vi "Right Motor Control Loop (SubVI).vi"   [LabVIEW 2015]
uses:
  Right Variables.vi
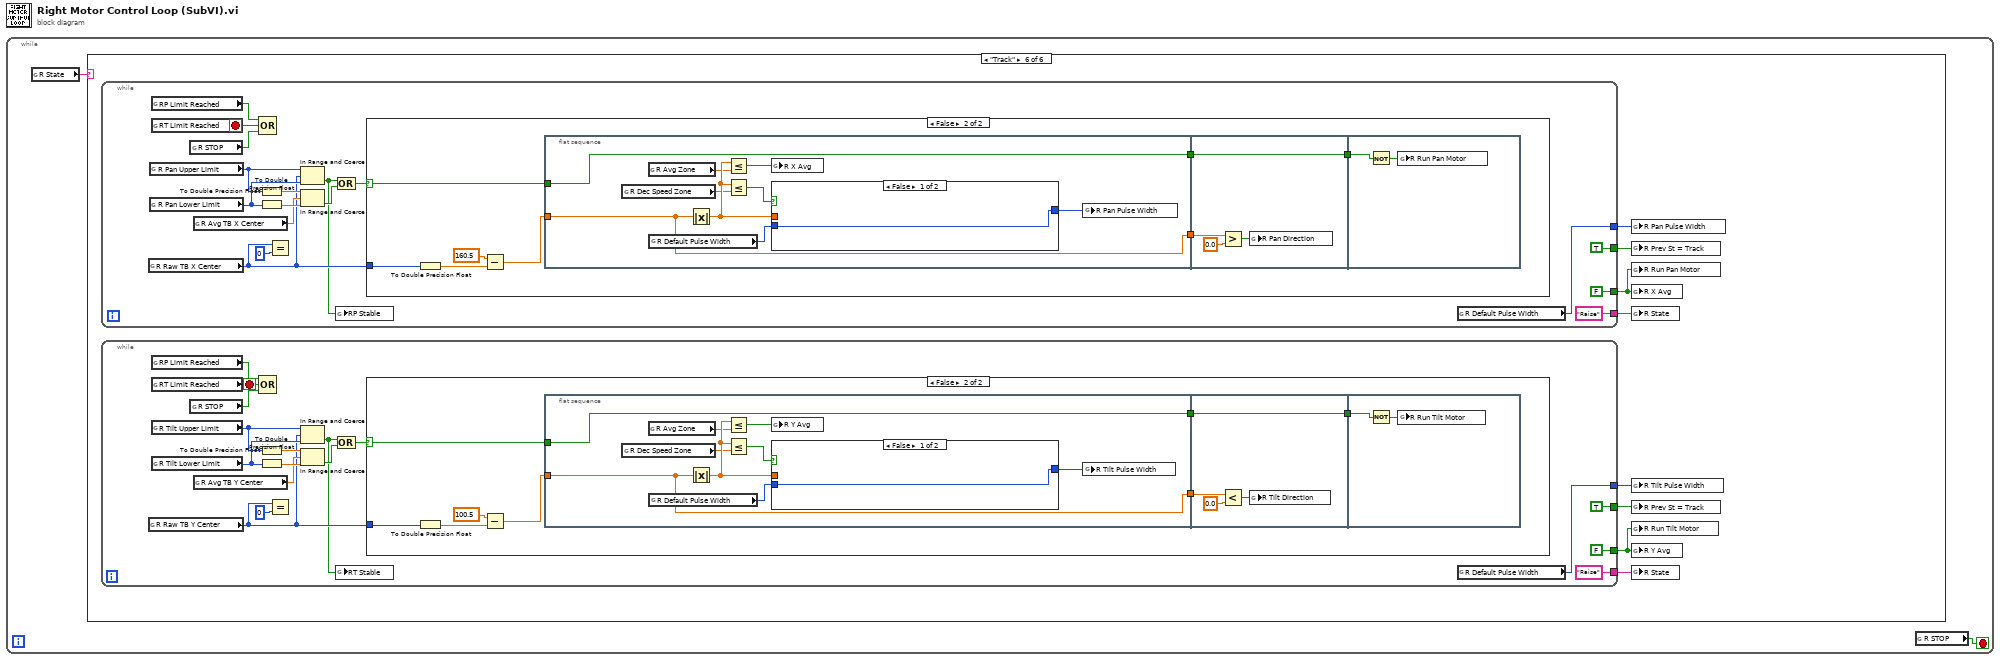
[diagram p0: block diagram]
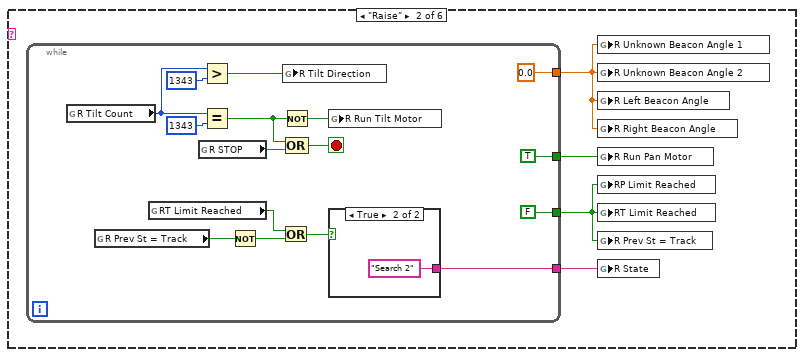
[diagram p3: hidden frame]
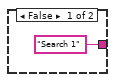
[diagram p4: hidden frame]
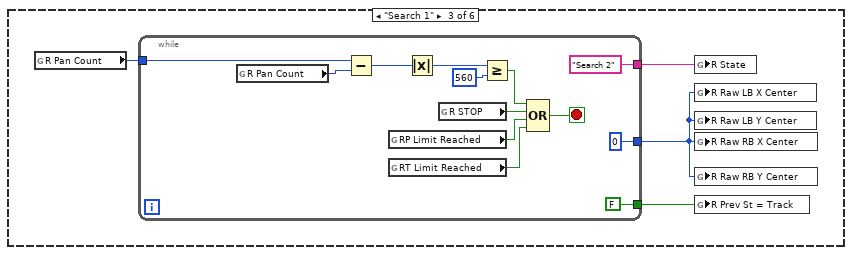
[diagram p5: hidden frame]
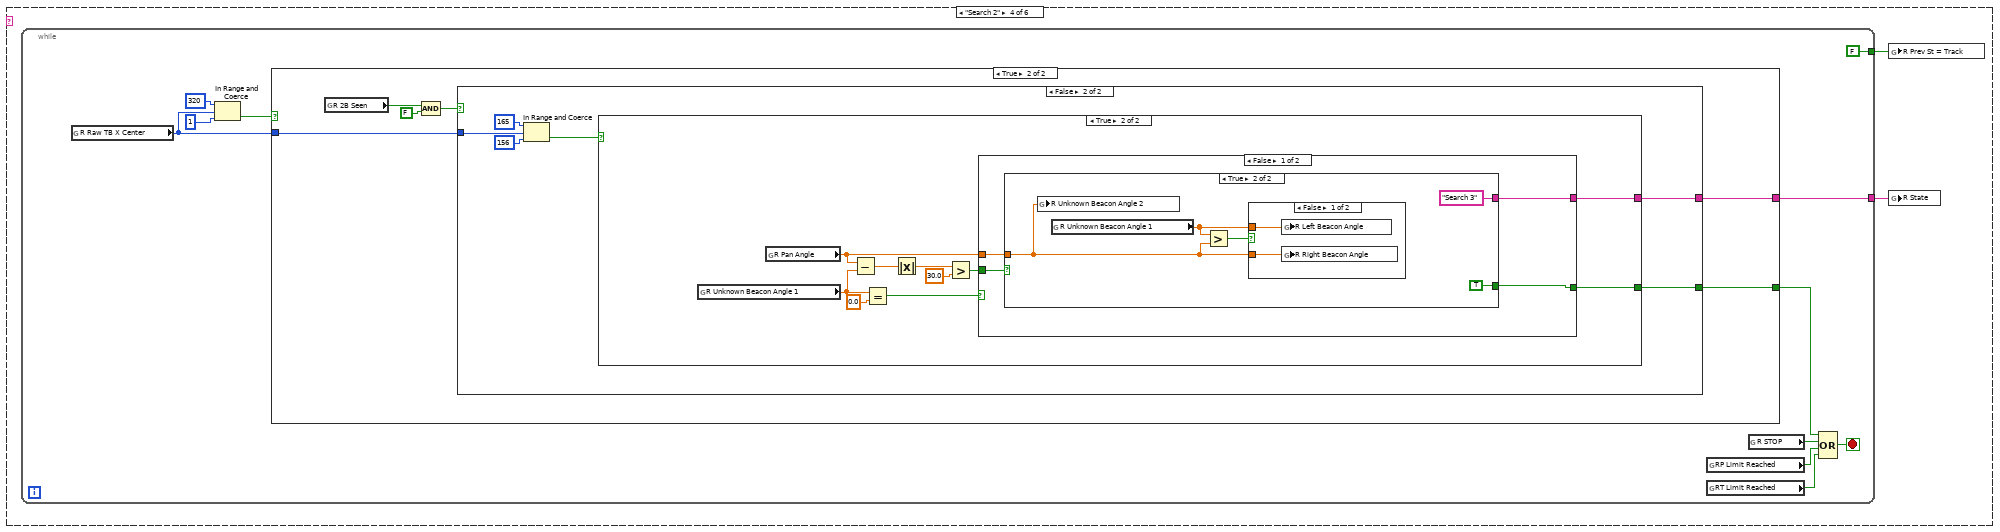
[diagram p6: hidden frame]
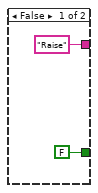
[diagram p7: hidden frame]
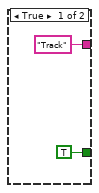
[diagram p8: hidden frame]
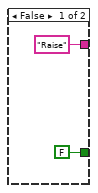
[diagram p9: hidden frame]
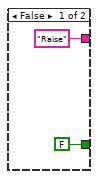
[diagram p10: hidden frame]
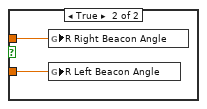
[diagram p11: hidden frame]
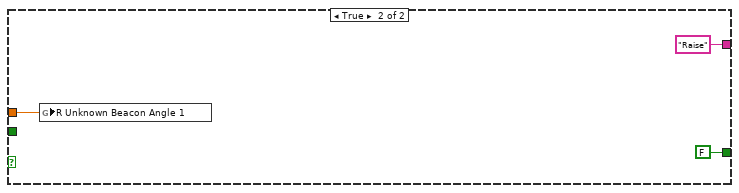
[diagram p12: hidden frame]
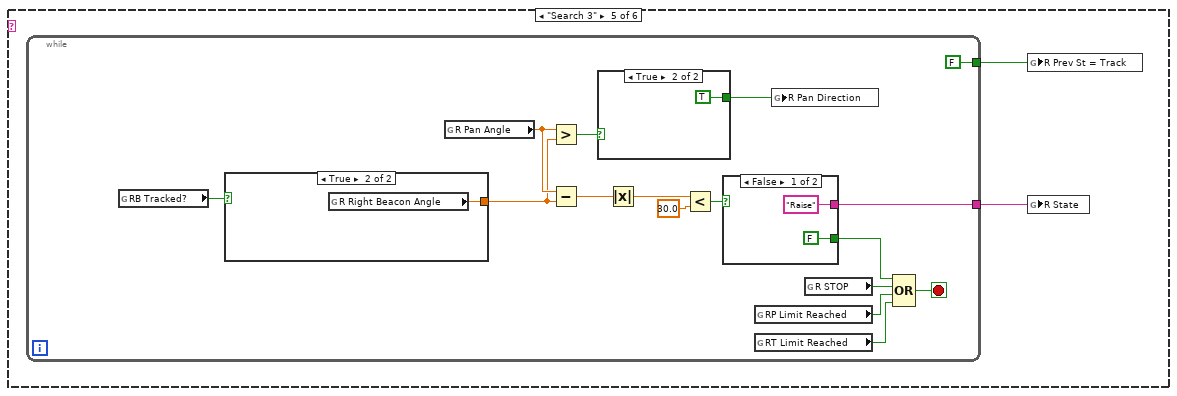
[diagram p13: hidden frame]
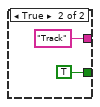
[diagram p14: hidden frame]
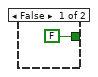
[diagram p15: hidden frame]
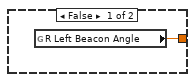
[diagram p16: hidden frame]
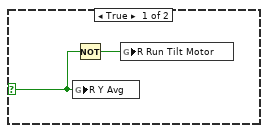
[diagram p17: hidden frame]
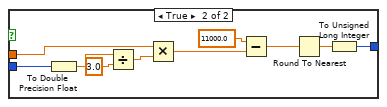
[diagram p18: hidden frame]
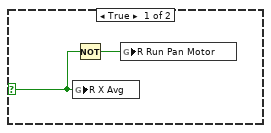
[diagram p19: hidden frame]
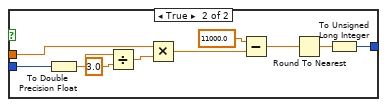
[diagram p20: hidden frame]
diagram:
  n1 = while {
    stop <- w1 stop-if-true
    n2 = global read "Right Variables.vi" "R State"() -> (w2:string)
    n3 = case shown="\"Track\"" w2 {
      frame "Null", Default {
      }
      frame "Raise" {
        n4 = while {
          tunnel: [w21] -> w6
          tunnel: [FALSE] -> w3
          tunnel: [TRUE ("L Run Pan Motor")] -> w5
          tunnel: [0.0] -> w4
          stop <- w22 stop-if-true
          n5 = global read "Right Variables.vi" "R Tilt Count"() -> (w17:i32)
          n6 = global read "Right Variables.vi" "R Prev St = Track"() -> (w10:bool)
          n7 = global read "Right Variables.vi" "RT Limit Reached"() -> (w8:bool)
          n8 = global read "Right Variables.vi" "R STOP"() -> (w14:bool)
          n9 = Greater?(x=w17, y=1343) -> (0:w15:bool)
          n10 = Equal?(x=w17, y=1343) -> (x = y?=w18:bool)
          n11 = Not(x=w10) -> (.not. x?=w9:bool)
          n12 = Or(x=w8, y=w9) -> (x .or. y?=w7:bool)
          n13 = Not(x=w18) -> (.not. x?=w16:bool)
          n14 = global write "Right Variables.vi" "R Tilt Direction"(w15) -> ()
          n15 = Compound Arithmetic op=OR(w18, w14) -> (w22:bool)
          n16 = global write "Right Variables.vi" "R Run Tilt Motor"(w16) -> ()
          n17 = case shown="True" w7 {
            tunnel: ["Search 1" ("L State") "Search 2" ("L State")] -> w21
            frame False {
            }
            frame True {
            }
          }
        }
        n18 = global write "Right Variables.vi" "R Unknown Beacon Angle 1"(w4) -> ()
        n19 = global write "Right Variables.vi" "R Unknown Beacon Angle 2"(w4) -> ()
        n20 = global write "Right Variables.vi" "R Left Beacon Angle"(w4) -> ()
        n21 = global write "Right Variables.vi" "R Right Beacon Angle"(w4) -> ()
        n22 = global write "Right Variables.vi" "R Run Pan Motor"(w5) -> ()
        n23 = global write "Right Variables.vi" "RP Limit Reached"(w3) -> ()
        n24 = global write "Right Variables.vi" "RT Limit Reached"(w3) -> ()
        n25 = global write "Right Variables.vi" "R Prev St = Track"(w3) -> ()
        n26 = global write "Right Variables.vi" "R State"(w6) -> ()
      }
      frame "Search 1" {
        n27 = global read "Right Variables.vi" "R Pan Count"() -> (w28:i32)
        n28 = while {
          tunnel: ["Search 2"] -> w27
          tunnel: w28 -> [w37]
          tunnel: [u16 0] -> w26
          tunnel: [FALSE] -> w25
          stop <- w41 stop-if-true
          n29 = global read "Right Variables.vi" "R Pan Count"() -> (w34:i32)
          n30 = Subtract(x=w37, y=w34) -> (x-y=w36:i32)
          n31 = global read "Right Variables.vi" "RP Limit Reached"() -> (w31:bool)
          n32 = global read "Right Variables.vi" "RT Limit Reached"() -> (w30:bool)
          n33 = Absolute Value(x=w36) -> (abs(x)=w35:i32)
          n34 = global read "Right Variables.vi" "R STOP"() -> (w33:bool)
          n35 = Greater Or Equal?(x=w35, y=560) -> (x >= y?=w38:bool)
          n36 = Compound Arithmetic op=OR(w38, w33, w31, w30) -> (w41:bool)
        }
        n37 = global write "Right Variables.vi" "R State"(w27) -> ()
        n38 = global write "Right Variables.vi" "R Raw LB X Center"(w26) -> ()
        n39 = global write "Right Variables.vi" "R Raw LB Y Center"(w26) -> ()
        n40 = global write "Right Variables.vi" "R Raw RB X Center"(w26) -> ()
        n41 = global write "Right Variables.vi" "R Raw RB Y Center"(w26) -> ()
        n42 = global write "Right Variables.vi" "R Prev St = Track"(w25) -> ()
      }
      frame "Search 2" {
        n43 = while {
          tunnel: [w48] -> w43
          tunnel: [FALSE] -> w42
          stop <- w52 stop-if-true
          n44 = global read "Right Variables.vi" "R Raw TB X Center"() -> (w49:u16)
          n45 = In Range and Coerce(upper limit=u16 320, x=w49, lower limit=u16 1) -> (In Range?=w50:bool)  [unwired: 1 out]
          n46 = case shown="True" w50 {
            tunnel: w49 -> [_ w62]
            tunnel: ["Raise" w61] -> w48
            tunnel: [FALSE w60] -> w47
            frame False {
            }
            frame True {
              n47 = global read "Right Variables.vi" "R 2B Seen"() -> (w59:bool)
              n48 = Compound Arithmetic op=AND(w59, FALSE ("y")) -> (w57:bool)
              n49 = case shown="False" w57 {
                tunnel: w62 -> [_ w70]
                tunnel: ["Track" w66] -> w61
                tunnel: [TRUE w67] -> w60
                frame True {
                }
                frame False {
                  n50 = In Range and Coerce(upper limit=u16 165, x=w70, lower limit=u16 156) -> (In Range?=w68:bool)  [unwired: 1 out]
                  n51 = case shown="True" w68 {
                    tunnel: [FALSE w76] -> w67
                    tunnel: ["Raise" w74] -> w66
                    frame False {
                    }
                    frame True {
                      n52 = global read "Right Variables.vi" "R Unknown Beacon Angle 1"() -> (w75:dbl)
                      n53 = global read "Right Variables.vi" "R Pan Angle"() -> (w73:dbl)
                      n54 = Subtract(x=w73, y=w75) -> (x-y=w81:dbl)
                      n55 = Equal?(x=w75, y=0.0) -> (x = y?=w78:bool)
                      n56 = Absolute Value(x=w81) -> (abs(x)=w80:dbl)
                      n57 = Greater?(x=w80, y=30.0) -> (0:w77:bool)
                      n58 = case shown="False" w78 {
                        tunnel: w73 -> [w86 w99]
                        tunnel: w77 -> [w85 _]
                        tunnel: [w84 FALSE] -> w76
                        tunnel: [w83 "Raise"] -> w74
                        frame False {
                          n59 = case shown="True" w85 {
                            tunnel: w86 -> [_ w89]
                            tunnel: [FALSE TRUE] -> w84
                            tunnel: ["Raise" "Search 3"] -> w83
                            frame False {
                            }
                            frame True {
                              n60 = global write "Right Variables.vi" "R Unknown Beacon Angle 2"(w89) -> ()
                              n61 = global read "Right Variables.vi" "R Unknown Beacon Angle 1"() -> (w91:dbl)
                              n62 = Greater?(x=w91, y=w89) -> (0:w93:bool)
                              n63 = case shown="False" w93 {
                                tunnel: w91 -> [w95 w97]
                                tunnel: w89 -> [w94 w96]
                                frame False {
                                n64 = global write "Right Variables.vi" "R Left Beacon Angle"(w95) -> ()
                                n65 = global write "Right Variables.vi" "R Right Beacon Angle"(w94) -> ()
                                }
                                frame True {
                                n66 = global write "Right Variables.vi" "R Right Beacon Angle"(w97) -> ()
                                n67 = global write "Right Variables.vi" "R Left Beacon Angle"(w96) -> ()
                                }
                              }
                            }
                          }
                        }
                        frame True {
                          n68 = global write "Right Variables.vi" "R Unknown Beacon Angle 1"(w99) -> ()
                        }
                      }
                    }
                  }
                }
              }
            }
          }
          n69 = global read "Right Variables.vi" "RP Limit Reached"() -> (w46:bool)
          n70 = global read "Right Variables.vi" "RT Limit Reached"() -> (w45:bool)
          n71 = global read "Right Variables.vi" "R STOP"() -> (w51:bool)
          n72 = Compound Arithmetic op=OR(w47, w51, w46, w45) -> (w52:bool)
        }
        n73 = global write "Right Variables.vi" "R Prev St = Track"(w42) -> ()
        n74 = global write "Right Variables.vi" "R State"(w43) -> ()
      }
      frame "Search 3" {
        n75 = while {
          tunnel: [w104] -> w102
          tunnel: [FALSE] -> w101
          stop <- w109 stop-if-true
          n76 = global read "Right Variables.vi" "RB Tracked?"() -> (w118:bool)
          n77 = case shown="True" w118 {
            tunnel: [w125 w126] -> w114
            frame False {
              n78 = global read "Right Variables.vi" "R Left Beacon Angle"() -> (w125:dbl)
            }
            frame True {
              n79 = global read "Right Variables.vi" "R Right Beacon Angle"() -> (w126:dbl)
            }
          }
          n80 = global read "Right Variables.vi" "R Pan Angle"() -> (w115:dbl)
          n81 = Greater?(x=w115, y=w114) -> (0:w117:bool)
          n82 = Subtract(x=w115, y=w114) -> (x-y=w106:dbl)
          n83 = case shown="True" w117 {
            tunnel: [FALSE TRUE] -> w116
            frame False {
            }
            frame True {
            }
          }
          n84 = Absolute Value(x=w106) -> (abs(x)=w105:dbl)
          n85 = Less?(x=w105, y=30.0) -> (x < y?=w112:bool)
          n86 = case shown="False" w112 {
            tunnel: ["Raise" "Track"] -> w104
            tunnel: [FALSE TRUE] -> w111
            frame False {
            }
            frame True {
            }
          }
          n87 = global read "Right Variables.vi" "RP Limit Reached"() -> (w108:bool)
          n88 = global read "Right Variables.vi" "RT Limit Reached"() -> (w107:bool)
          n89 = global write "Right Variables.vi" "R Pan Direction"(w116) -> ()
          n90 = global read "Right Variables.vi" "R STOP"() -> (w110:bool)
          n91 = Compound Arithmetic op=OR(w111, w110, w108, w107) -> (w109:bool)
        }
        n92 = global write "Right Variables.vi" "R Prev St = Track"(w101) -> ()
        n93 = global write "Right Variables.vi" "R State"(w102) -> ()
      }
      frame "Track" {
        n94 = while {
          tunnel: ["Raise"] -> w134
          tunnel: [FALSE] -> w131
          tunnel: [TRUE] -> w130
          tunnel: [w189] -> w128
          stop <- w206 stop-if-true
          n95 = global read "Right Variables.vi" "R Raw TB X Center"() -> (w194:u16)
          n96 = global read "Right Variables.vi" "R Pan Upper Limit"() -> (w201:u16)
          n97 = global read "Right Variables.vi" "R Pan Lower Limit"() -> (w200:u16)
          n98 = global read "Right Variables.vi" "RP Limit Reached"() -> (w196:bool)
          n99 = global read "Right Variables.vi" "RT Limit Reached"() -> (w198:bool)
          n100 = global read "Right Variables.vi" "R STOP"() -> (w197:bool)
          n101 = global read "Right Variables.vi" "R Avg TB X Center"() -> (w199:dbl)
          n102 = Compound Arithmetic op=OR(w196, w198, w197) -> (w206:bool)
          n103 = To Double Precision Float(number=w201) -> (double precision float=w204:dbl)
          n104 = To Double Precision Float(number=w200) -> (double precision float=w203:dbl)
          n105 = Equal?(x=w194, y=u16 0) -> ()  [unwired: 1 out]
          n106 = In Range and Coerce(upper limit=w201, x=w194, lower limit=w200) -> (In Range?=w192:bool)  [unwired: 1 out]
          n107 = In Range and Coerce(upper limit=w204, x=w199, lower limit=w203) -> (In Range?=w202:bool)  [unwired: 1 out]
          n108 = global write "Right Variables.vi" "RP Stable"(w192) -> ()
          n109 = Compound Arithmetic op=OR(w192, w202) -> (w191:bool)
          n110 = case shown="False" w191 {
            selector: w191 -> [w208 w209]
            tunnel: w194 -> [_ w216]
            frame True {
              n111 = global write "Right Variables.vi" "R X Avg"(w208) -> ()
              n112 = Not(x=w208) -> (.not. x?=w207:bool)
              n113 = global write "Right Variables.vi" "R Run Pan Motor"(w207) -> ()
            }
            frame False {
              n114 = To Double Precision Float(number=w216) -> (double precision float=w214:dbl)
              n115 = Subtract(x=160.5, y=w214) -> (x-y=w213:dbl)
              n116 = flat-sequence {
                tunnel: w213 -> [w218]
                tunnel: [w218] -> w212
                tunnel: [w217] -> w210
                tunnel: w209 -> [w217]
                tunnel: w212 -> [w238]
                tunnel: [w237] -> w211
                tunnel: w210 -> [w237]
                tunnel: w211 -> [w241]
                frame #0 {
                  n117 = global read "Right Variables.vi" "R Dec Speed Zone"() -> (w222:dbl)
                  n118 = global read "Right Variables.vi" "R Avg Zone"() -> (w223:dbl)
                  n119 = global read "Right Variables.vi" "R Default Pulse Width"() -> (w221:u32)
                  n120 = Absolute Value(x=w218) -> (abs(x)=w224:dbl)
                  n121 = Less Or Equal?(x=w224, y=w223) -> (x <= y?=w220:bool)
                  n122 = Less Or Equal?(x=w224, y=w222) -> (x <= y?=w225:bool)
                  n123 = global write "Right Variables.vi" "R X Avg"(w220) -> ()
                  n124 = case shown="False" w225 {
                    tunnel: w221 -> [w226 w236]
                    tunnel: [w226 w229] -> w219
                    tunnel: w224 -> [_ w227]
                    frame False {
                    }
                    frame True {
                      n125 = To Double Precision Float(number=w236) -> (double precision float=w228:dbl)
                      n126 = Divide(x=w228, y=3.0) -> (x/y=w233:dbl)
                      n127 = Multiply(x=w227, y=w233) -> (x*y=w232:dbl)
                      n128 = Subtract(x=11000.0, y=w232) -> (x-y=w231:dbl)
                      n129 = Round To Nearest(number=w231) -> (nearest integer value=w230:dbl)
                      n130 = To Unsigned Long Integer(number=w230) -> (unsigned 32bit integer=w229:u32)
                    }
                  }
                  n131 = global write "Right Variables.vi" "R Pan Pulse Width"(w219) -> ()
                }
                frame #1 {
                  n132 = Greater?(x=w238, y=0.0) -> (0:w240:bool)
                  n133 = global write "Right Variables.vi" "R Pan Direction"(w240) -> ()
                }
                frame #2 {
                  n134 = Not(x=w241) -> (.not. x?=w242:bool)
                  n135 = global write "Right Variables.vi" "R Run Pan Motor"(w242) -> ()
                }
              }
            }
          }
          n136 = global read "Right Variables.vi" "R Default Pulse Width"() -> (w189:u32)
        }
        n137 = while {
          tunnel: ["Raise"] -> w133
          tunnel: [FALSE] -> w132
          tunnel: [TRUE] -> w129
          tunnel: [w135] -> w127
          stop <- w152 stop-if-true
          n138 = global read "Right Variables.vi" "R Raw TB Y Center"() -> (w139:u16)
          n139 = global read "Right Variables.vi" "RP Limit Reached"() -> (w142:bool)
          n140 = global read "Right Variables.vi" "RT Limit Reached"() -> (w146:bool)
          n141 = global read "Right Variables.vi" "R Tilt Upper Limit"() -> (w145:u16)
          n142 = global read "Right Variables.vi" "R Tilt Lower Limit"() -> (w144:u16)
          n143 = global read "Right Variables.vi" "R STOP"() -> (w147:bool)
          n144 = global read "Right Variables.vi" "R Avg TB Y Center"() -> (w143:dbl)
          n145 = Compound Arithmetic op=OR(w142, w146, w147) -> (w152:bool)
          n146 = To Double Precision Float(number=w145) -> (double precision float=w150:dbl)
          n147 = To Double Precision Float(number=w144) -> (double precision float=w149:dbl)
          n148 = Equal?(x=w139, y=u16 0) -> ()  [unwired: 1 out]
          n149 = In Range and Coerce(upper limit=w145, x=w139, lower limit=w144) -> (In Range?=w138:bool)  [unwired: 1 out]
          n150 = In Range and Coerce(upper limit=w150, x=w143, lower limit=w149) -> (In Range?=w148:bool)  [unwired: 1 out]
          n151 = global write "Right Variables.vi" "RT Stable"(w138) -> ()
          n152 = Compound Arithmetic op=OR(w138, w148) -> (w137:bool)
          n153 = case shown="False" w137 {
            selector: w137 -> [w154 w155]
            tunnel: w139 -> [_ w162]
            frame True {
              n154 = global write "Right Variables.vi" "R Y Avg"(w154) -> ()
              n155 = Not(x=w154) -> (.not. x?=w153:bool)
              n156 = global write "Right Variables.vi" "R Run Tilt Motor"(w153) -> ()
            }
            frame False {
              n157 = To Double Precision Float(number=w162) -> (double precision float=w160:dbl)
              n158 = Subtract(x=100.5, y=w160) -> (x-y=w159:dbl)
              n159 = flat-sequence {
                tunnel: w159 -> [w164]
                tunnel: [w164] -> w158
                tunnel: [w163] -> w156
                tunnel: w155 -> [w163]
                tunnel: w158 -> [w184]
                tunnel: [w183] -> w157
                tunnel: w156 -> [w183]
                tunnel: w157 -> [w187]
                frame #0 {
                  n160 = global read "Right Variables.vi" "R Dec Speed Zone"() -> (w166:dbl)
                  n161 = global read "Right Variables.vi" "R Avg Zone"() -> (w167:dbl)
                  n162 = global read "Right Variables.vi" "R Default Pulse Width"() -> (w168:u32)
                  n163 = Absolute Value(x=w164) -> (abs(x)=w170:dbl)
                  n164 = Less Or Equal?(x=w170, y=w167) -> (x <= y?=w165:bool)
                  n165 = Less Or Equal?(x=w170, y=w166) -> (x <= y?=w171:bool)
                  n166 = global write "Right Variables.vi" "R Y Avg"(w165) -> ()
                  n167 = case shown="False" w171 {
                    tunnel: w168 -> [w172 w176]
                    tunnel: [w172 w175] -> w169
                    tunnel: w170 -> [_ w173]
                    frame False {
                    }
                    frame True {
                      n168 = To Double Precision Float(number=w176) -> (double precision float=w174:dbl)
                      n169 = Divide(x=w174, y=3.0) -> (x/y=w179:dbl)
                      n170 = Multiply(x=w173, y=w179) -> (x*y=w180:dbl)
                      n171 = Subtract(x=11000.0, y=w180) -> (x-y=w181:dbl)
                      n172 = Round To Nearest(number=w181) -> (nearest integer value=w182:dbl)
                      n173 = To Unsigned Long Integer(number=w182) -> (unsigned 32bit integer=w175:u32)
                    }
                  }
                  n174 = global write "Right Variables.vi" "R Tilt Pulse Width"(w169) -> ()
                }
                frame #1 {
                  n175 = Less?(x=w184, y=0.0) -> (x < y?=w186:bool)
                  n176 = global write "Right Variables.vi" "R Tilt Direction"(w186) -> ()
                }
                frame #2 {
                  n177 = Not(x=w187) -> (.not. x?=w188:bool)
                  n178 = global write "Right Variables.vi" "R Run Tilt Motor"(w188) -> ()
                }
              }
            }
          }
          n179 = global read "Right Variables.vi" "R Default Pulse Width"() -> (w135:u32)
        }
        n180 = global write "Right Variables.vi" "R Pan Pulse Width"(w128) -> ()
        n181 = global write "Right Variables.vi" "R Prev St = Track"(w130) -> ()
        n182 = global write "Right Variables.vi" "R Run Pan Motor"(w131) -> ()
        n183 = global write "Right Variables.vi" "R X Avg"(w131) -> ()
        n184 = global write "Right Variables.vi" "R State"(w134) -> ()
        n185 = global write "Right Variables.vi" "R Tilt Pulse Width"(w127) -> ()
        n186 = global write "Right Variables.vi" "R Prev St = Track"(w129) -> ()
        n187 = global write "Right Variables.vi" "R Run Tilt Motor"(w132) -> ()
        n188 = global write "Right Variables.vi" "R Y Avg"(w132) -> ()
        n189 = global write "Right Variables.vi" "R State"(w133) -> ()
      }
    }
    n190 = global read "Right Variables.vi" "R STOP"() -> (w1:bool)
  }
